vi "PC_DPG to DPWMM.vi"() -> ()   [LabVIEW 2021]
uses:
  Digital PWM Measurement/Typedefs/Digital PWM Measurements.ctl
  Digital Pulse Generation/Typedefs/Digital Pulse Settings.ctl
  Digital Pulse Generation/Typedefs/Actual Pulse Settings.ctl
  Common/Typedefs/Execution Options - Measure.ctl
  Digital PWM Measurement/DAQ_Digital PWM Measurement.lvlib
  Digital Pulse Generation/DAQ_Digital Pulse Generation.lvlib
panel:
  out "Actual Pulse Settings":T1={"High Time (s)"=0.0015, "Low Time (s)"=0.0005, "Generation Time (s)"=0.008} {"Low Time (s)" format="%.2p"; "High Time (s)" format="%.2p"; "Generation Time (s)" format="%.2p"}
  in  "Digital Pulse Settings":T2={"High Time (s)"=0.0015, "Low Time (s)"=0.0005, "Number of Pulses"=4} {"Low Time (s)" format="%.2p"; "High Time (s)" format="%.2p"}
  out "Digital PWM Measurements":T3={"High Time (s)"=0.0015000000000000002, "Low Time (s)"=0.0005, "Duty Cycle (%)"=75.00000000000001, "Frequency (Hz)"=500.0} {"Frequency (Hz)" format="%.6p"; "Duty Cycle (%)" min=0.0 max=100.0 format="%#.2p"; "Low Time (s)" format="%.2p"; "High Time (s)" format="%.2p"}
  out "Actual Cycles Captured":i32=4
  in  "Cycles to capture":i32=4 min=2 step=1
  out "error out":errorcluster
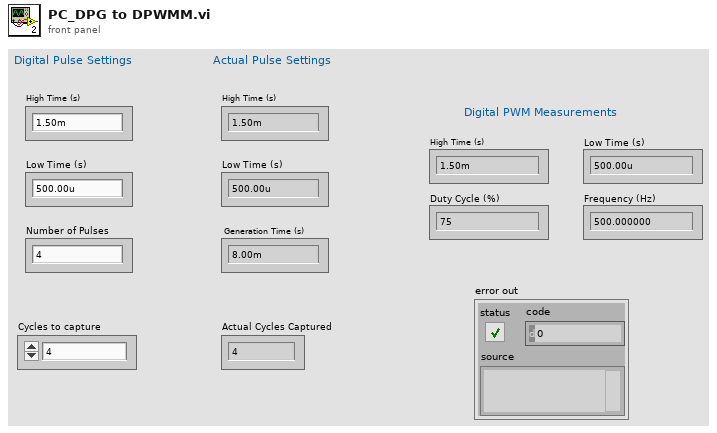
[diagram p1: front panel]
types:
  T1 = typedef "DAQ_Digital Pulse Generation.lvlib/Actual Pulse Settings.ctl" = cluster{"High Time (s)":dbl, "Low Time (s)":dbl, "Generation Time (s)":dbl}
  T2 = typedef "DAQ_Digital Pulse Generation.lvlib/Digital Pulse Settings.ctl" = cluster{"High Time (s)":dbl, "Low Time (s)":dbl, "Number of Pulses":i32}
  T3 = typedef "DAQ_Digital PWM Measurement.lvlib/Digital PWM Measurements.ctl" = cluster{"High Time (s)":dbl, "Low Time (s)":dbl, "Duty Cycle (%)":dbl, "Frequency (Hz)":dbl}
  T4 = typedef "Execution Options - Measure.ctl" = enum16{"Configure & Measure", "Configure only", "Measure only"}
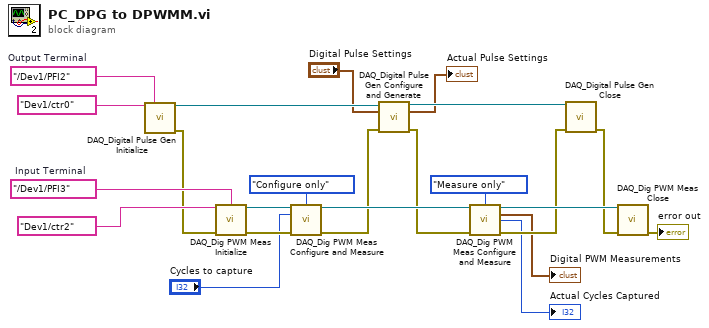
[diagram p0: block diagram]
diagram:
  w21 = tag "/Dev1/PFI3"  # Input Terminal
  w19 = tag "/Dev1/PFI2"  # Output Terminal
  n1 = call "DAQ_Digital Pulse Gen Initialize.vi"("Physical Channel (Counter)"=tag "Dev1/ctr0", "Output Terminal"=w19) -> ("DAQmx Task Out"=w15:refnum<k21>, "error out"=w20:errorcluster)  [unwired: 12 in]
  n2 = call "DAQ_Dig PWM Meas Initialize.vi"("Physical Channel (counter)"=tag "Dev1/ctr2", "Input Terminal"=w21, "error in"=w20) -> ("DAQmx Task Out"=w18:refnum<k21>, "error out"=w13:errorcluster)  [unwired: 11 in]
  n3 = call "DAQ_Dig PWM Meas Configure and Measure.vi"("DAQmx Task In"=w18, "Execution Option"=Execution_Options_-_Measure."Configure only", "Cycles to capture"="Cycles to capture", "error in"=w13) -> ("DAQmx Task Out"=w17:refnum<k21>, "error out"=w12:errorcluster)  [unwired: 8 in, 2 out]
  n4 = call "DAQ_Digital Pulse Gen Configure and Generate.vi"("DAQmx Task In"=w15, "Digital Pulse Settings"="Digital Pulse Settings", "error in"=w12) -> ("DAQmx Task Out"=w14:refnum<k21>, "Actual Pulse Settings"=→"Actual Pulse Settings":T1, "error out"=w11:errorcluster)  [unwired: 10 in]
  n5 = call "DAQ_Dig PWM Meas Configure and Measure.vi"("DAQmx Task In"=w17, "Execution Option"=Execution_Options_-_Measure."Measure only", "error in"=w11) -> ("DAQmx Task Out"=w16:refnum<k21>, "Digital PWM Measurements"=→"Digital PWM Measurements":T3, "Actual Cycles Captured"=→"Actual Cycles Captured":i32, "error out"=w10:errorcluster)  [unwired: 9 in]
  n6 = call "DAQ_Digital Pulse Gen Close.vi"("DAQmx Task In"=w14, "error in"=w10) -> ("error out"=w9:errorcluster)  [unwired: 13 in]
  n7 = call "DAQ_Dig PWM Meas Close.vi"("DAQmx Task In"=w16, "error in"=w9) -> ("error out"=→"error out":errorcluster)  [unwired: 13 in]
